vi "Send.vi"(4 "Is Priority":bool, 6 "Self Attributes":T3, 8 "Relation":T2=enum."Created", 9 "Msg":refnum<class "Msg.lvclass">, 10 "Attributes":T3) -> (2 "Error Info":T1)   [LabVIEW 2020, in "jettl.lvlib" / "Actor.lvlib" / "Base Actor.lvclass"]
uses:
  Base Actor.lvclass
  Attributes.ctl
  Msg/Msg.lvclass
  Implemented Msgs.ctl
  Relation.ctl
  Error Info.ctl
  <vilib>/event_ctls.llb/usereventprio.ctl
  Sender/Sender/Sender.lvclass
  Sender/Sender.lvlib
  Actor.lvlib
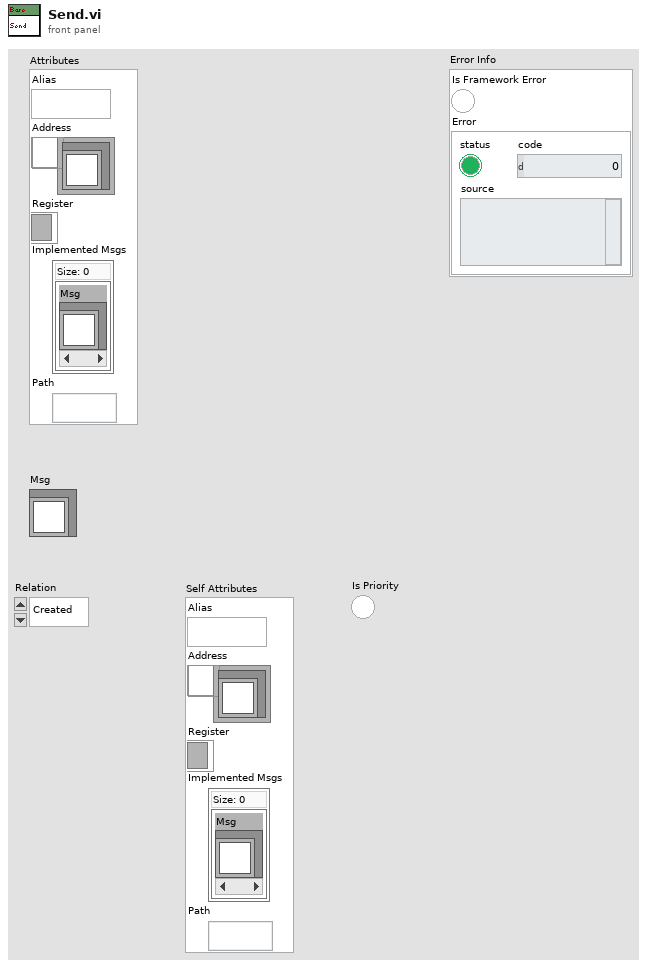
[diagram p1: front panel]
types:
  T1 = typedef "jettl.lvlib/Actor.lvlib/Error Info.ctl" = cluster{"Is Framework Error":bool, "Error":errorcluster}
  T2 = typedef "jettl.lvlib/Actor.lvlib/Relation.ctl" = enum16{"Self", "Creator", "Created"}
  T3 = typedef "jettl.lvlib/Actor.lvlib/Attributes.ctl" = cluster{"Alias":string, "Address":refnum<user-event>, "Register":refnum<event-registration>, "Implemented Msgs":T4, "Path":path}
  T4 = typedef "jettl.lvlib/Actor.lvlib/Implemented Msgs.ctl" = set{refnum<class "Msg.lvclass">}
  T5 = typedef "usereventprio.ctl" = enum32{"high priority", "normal priority"}
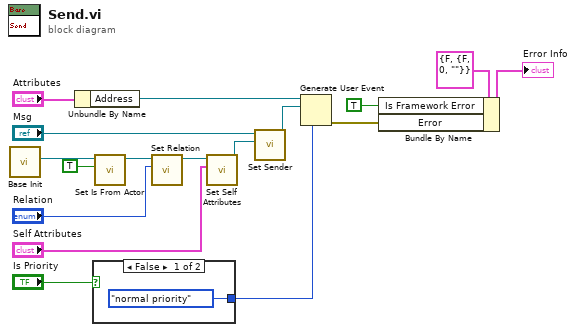
[diagram p0: block diagram]
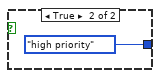
[diagram p2: hidden frame]
diagram:
  n1 = call "Base Init.vi"() -> ("Sender"=w9:refnum<class "Sender.lvclass">)  [unwired: 11 in]
  n2 = Unbundle By Name("Attributes") -> ("Address"=w15:refnum<user-event>)
  n3 = case shown="False" "Is Priority" {
    tunnel: [usereventprio."normal priority" ("priority (normal)") usereventprio."high priority" ("priority (normal)")] -> w16
    frame False {
    }
    frame True {
    }
  }
  n4 = call-dynamic "Set Is From Actor.vi"("Is From Actor"=TRUE, "Sender in"=w9) -> ("Sender out"=w11:refnum<class "Sender.lvclass">)  [unwired: 9 in]
  n5 = call-dynamic "Set Relation.vi"("Relation"="Relation", "Sender in"=w11) -> ("Sender out"=w10:refnum<class "Sender.lvclass">)  [unwired: 9 in]
  n6 = call-dynamic "Set Self Attributes.vi"("Self Attributes"="Self Attributes", "Sender in"=w10) -> ("Sender out"=w12:refnum<class "Sender.lvclass">)  [unwired: 9 in]
  n7 = call-dynamic "Set Sender.vi"("Sender"=w12, "Msg in"="Msg") -> ("Msg out"=w7:refnum<class "Msg.lvclass">)  [unwired: 9 in]
  n8 = Generate User Event(priority (normal)=w16, user event=w15, event data cluster=w7) -> (error out=w1:errorcluster)  [unwired: 1 in, 1 out]
  n9 = Bundle By Name(cluster=T1 {"Is Framework Error"=FALSE, "Error"={"status"=FALSE, "code"=0, "source"=""}} ("Error Info"), "Is Framework Error"=TRUE, "Error"=w1) -> (→"Error Info":T1)
